vi "L_bank_driving.vi"(0 "MD403.lvclass":refnum<class "MD403.lvclass">, 1 "ACT-Ctrl ON":bool, 2 "NFL-Ctrl ON":bool, 3 "L-bank too high":bool, 4 "L too low":bool, 5 "error in":errorcluster, 6 "ACT Ctrl-Output":dbl, 7 "NFL Ctrl-Output":dbl) -> (8 "NFL/ ACT-C Auto":bool, 9 "NFL-/ ACT-Ctrl\nOutput signal":dbl, 14 "MD403.lvclass out":refnum<class "MD403.lvclass">, 15 "L ins Ctrl":u32, 16 "L fast Ctrl":bool, 17 "L withdr Ctrl":u32, 19 "error out":errorcluster)   [LabVIEW 2022 SP3, in "MD403.lvclass"]
uses:
  MD403.lvclass
  MD403.lvclass/MD403.ctl
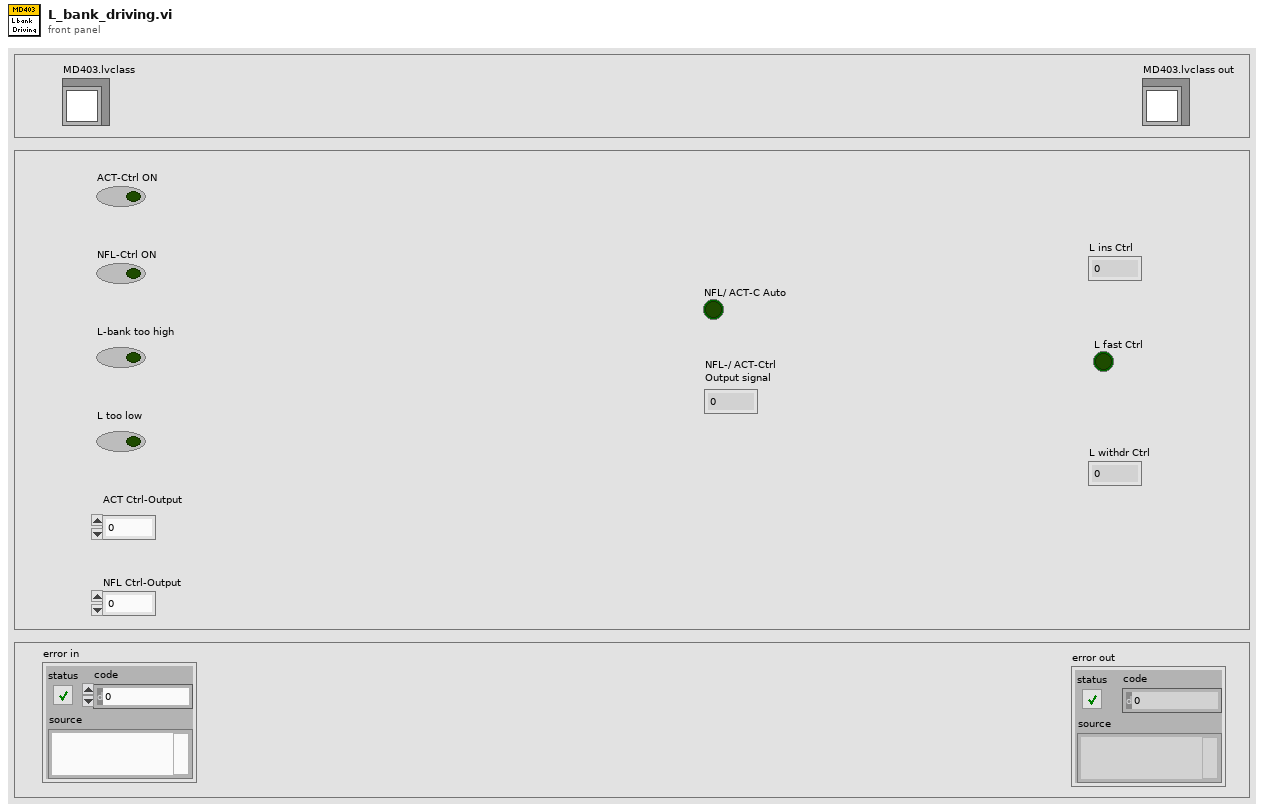
[diagram p1: front panel]
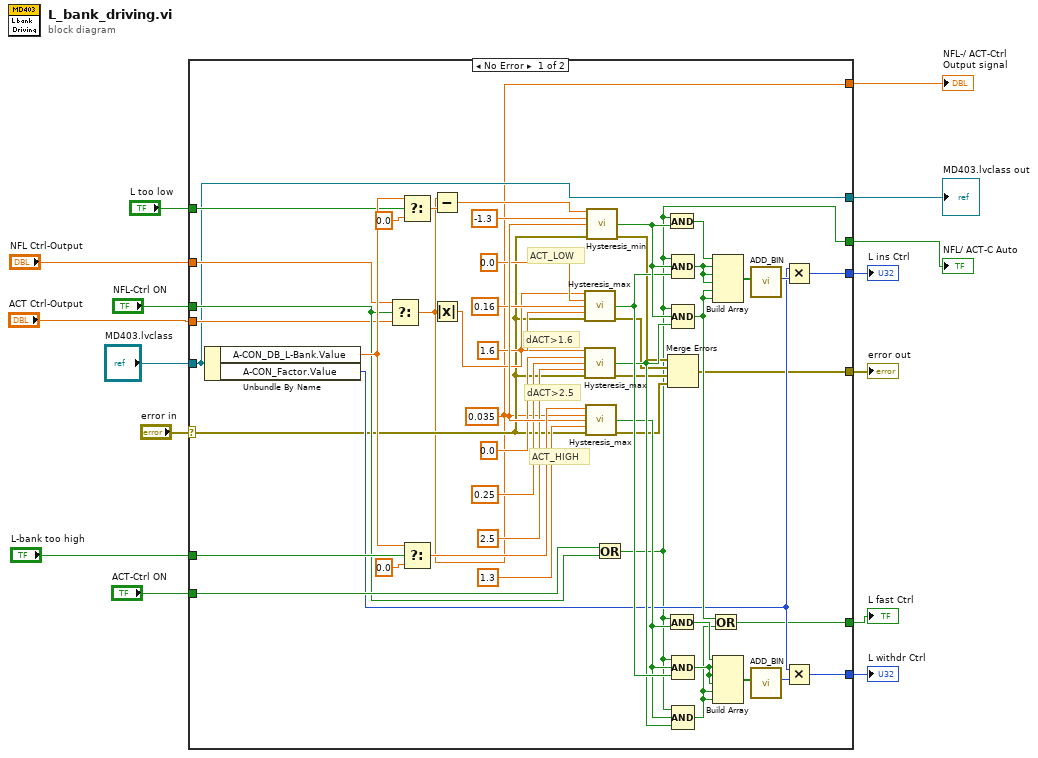
[diagram p0: block diagram]
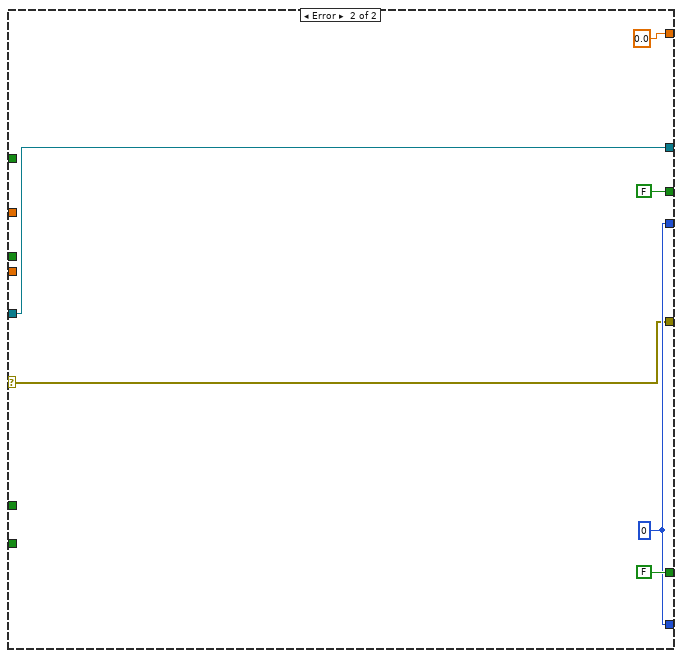
[diagram p2: hidden frame]
diagram:
  n1 = case shown="No Error" "error in" {
    selector: "error in" -> [w23 w68]
    tunnel: "ACT-Ctrl ON" -> [w59 _]
    tunnel: "NFL-Ctrl ON" -> [w58 _]
    tunnel: "L-bank too high" -> [w64 _]
    tunnel: "L too low" -> [w60 _]
    tunnel: "ACT Ctrl-Output" -> [w56 _]
    tunnel: "NFL Ctrl-Output" -> [w57 _]
    tunnel: "MD403.lvclass" -> [w24 w67]
    tunnel: [w27 w69] -> w7
    tunnel: [w26 w69] -> w6
    tunnel: [w25 FALSE] -> w5
    tunnel: [w24 w67] -> w4
    tunnel: [w18 w68] -> w3
    tunnel: [w17 FALSE] -> w2
    tunnel: [w16 0.0 ("ACT Ctrl-Output")] -> w1
    frame No Error {
      w52 = 0.035 ("H")
      # "dACT>2.5"
      # "dACT>1.6"
      # "ACT_LOW"
      # "ACT_HIGH"
      n2 = Unbundle By Name(w24) -> ("A-CON_DB_L-Bank.Value"=w62:dbl, "A-CON_Factor.Value"=w28:u32)
      n3 = Select(t=w57, s=w58, f=w56) -> (s? t:f=w16:dbl)
      n4 = Select(t=w62, s=w60, f=0.0) -> (s? t:f=w53:dbl)
      n5 = Select(t=w62, s=w64, f=0.0) -> (s? t:f=w55:dbl)
      n6 = Subtract(x=w16, y=w53) -> (x-y=w54:dbl)
      n7 = Absolute Value(x=w16) -> (abs(x)=w47:dbl)
      n8 = call "Hysteresis_max.vi"("input(+)"=w47, "input (-)"=0.0, "H"=0.16, "Max"=1.6, "error in"=w23) -> ("Deviation"=w41:bool, "error out"=w21:errorcluster)  [unwired: 9 in]
      n9 = call "Hysteresis_max.vi"("input(+)"=w47, "input (-)"=0.0, "H"=0.25, "Max"=2.5, "error in"=w23) -> ("Deviation"=w40:bool, "error out"=w20:errorcluster)  [unwired: 9 in]
      n10 = call "Hysteresis_max.vi"("input(+)"=w55, "input (-)"=w16, "H"=w52, "Max"=1.3, "error in"=w23) -> ("Deviation"=w39:bool, "error out"=w19:errorcluster)  [unwired: 9 in]
      n11 = call "Hysteresis_min.vi"("input"=w54, "Min"=-1.3, "H"=w52, "error in"=w23) -> ("Deviation"=w42:bool, "error out"=w22:errorcluster)  [unwired: 10 in]
      n12 = Or(x=w59, y=w58) -> (x .or. y?=w17:bool)
      n13 = And(x=w17, y=w42) -> (x .and. y?=w38:bool)
      n14 = And(x=w17, y=w39) -> (x .and. y?=w35:bool)
      n15 = Merge Errors(w22, w21, w20, w19) -> (w18:errorcluster)
      n16 = Compound Arithmetic op=AND(w17, w42, w41) -> (w37:bool)
      n17 = Compound Arithmetic op=AND(w17, w42, w40) -> (w32:bool)
      n18 = Compound Arithmetic op=AND(w17, w39, w41) -> (w34:bool)
      n19 = Compound Arithmetic op=AND(w17, w39, w40) -> (w31:bool)
      n20 = Or(x=w32, y=w31) -> (x .or. y?=w25:bool)
      n21 = Build Array(w38, w37, w37, w37, w32, w32) -> (w36:bool[])
      n22 = Build Array(w35, w34, w34, w34, w31, w31) -> (w33:bool[])
      n23 = call "ADD_BIN.vi"("Array"=w36) -> ("SUM"=w30:i16)  [unwired: 10 in]
      n24 = call "ADD_BIN.vi"("Array"=w33) -> ("SUM"=w29:i16)  [unwired: 10 in]
      n25 = Multiply(x=w28, y=w30) -> (x*y=w27:u32)
      n26 = Multiply(x=w28, y=w29) -> (x*y=w26:u32)
    }
    frame Error {
      w69 = u32 0
    }
  }
  "L ins Ctrl" <- w7
  "L withdr Ctrl" <- w6
  "L fast Ctrl" <- w5
  "MD403.lvclass out" <- w4
  "error out" <- w3
  "NFL/ ACT-C Auto" <- w2
  "NFL-/ ACT-Ctrl\nOutput signal" <- w1
